vi "BuildRunScript.vi"(8 "ErrorArray In":errorcluster[](array[cluster]), 11 "NISTBus In":refnum<class "NISTBus.lvclass">) -> (0 "ErrorArray Out":errorcluster[](array[cluster]), 2 "Script":string[](array[string]), 3 "NISTBus Out":refnum<class "NISTBus.lvclass">)   [LabVIEW 2014, in "TestFramework.lvlib"]
uses:
  TestFramework.lvlib
  Bus/NISTBus.lvclass
  FGenModule/PublicAPI/Arguments/Broadcasts/clErrorRpt.ctl
  FGenPlugins/MyPluginBaseClass/TypeDef/PluginParams.ctl
  WfrmGenerator/WfrmModule/PublicAPI/Arguments/Broadcasts/clErrorRpt.ctl
  WfrmGenerator/WfrmModule/PublicAPI/Arguments/Requests/clLoadPlugin.ctl
  <vilib>/Utility/error.llb/Error Cluster From Error Code.vi
  <vilib>/ErrorRing/Error Ring.xnode
  FGenModule/FGenModule.lvlib
  <userlib>/NIST/NISTErrorLib/NISTErrorLib.lvlib
  WfrmGenerator/WfrmModule/WfrmModule.lvlib
  FGenPlugins/MyPluginBaseClass/NISTFGenPluginsBase.lvclass
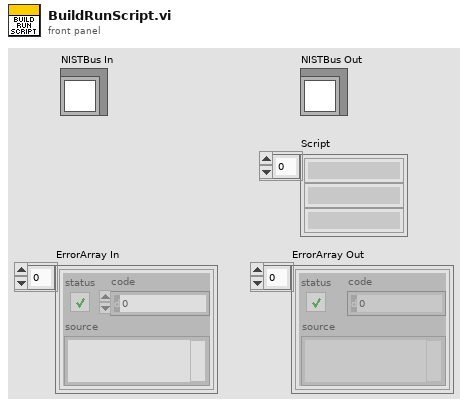
[diagram p1: front panel]
types:
  T1 = typedef "FGenModule.lvlib/clErrorRpt.ctl" = cluster{"error":errorcluster, "AdditionalInfo":string}
  T2 = typedef "WfrmModule.lvlib/clErrorRpt.ctl" = cluster{"error":errorcluster, "AdditionalInfo":string}
  T3 = typedef "WfrmModule.lvlib/clLoadPlugin.ctl" = cluster{"PathToPlugin":path}
  T4 = typedef "FGenModule.lvlib/clBroadcastEvents.ctl" = cluster{"DidInit":refnum<user-event>, "StatusUpdate":refnum<user-event>, "ErrorReport":refnum<user-event>, "DidStop":refnum<user-event>, "PathToINI":refnum<user-event>, "ChannelName":refnum<user-event>}
  T5 = typedef "FGenPlugins.lvlib/NISTFGenPluginsBase.lvclass/PluginParams.ctl" = cluster{"Path to Plugin INI":path}
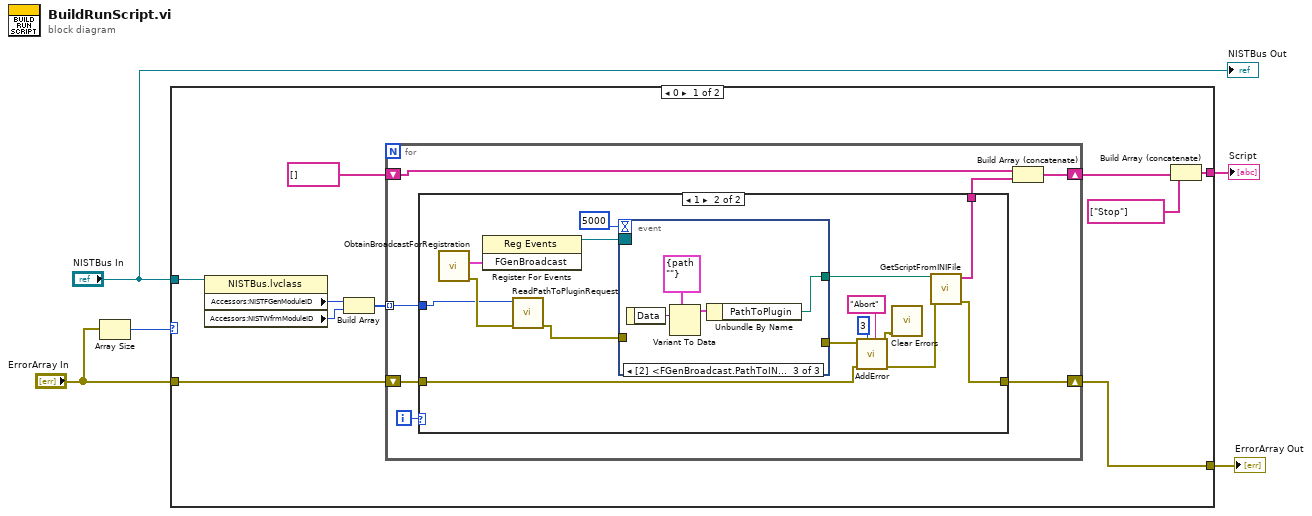
[diagram p0: block diagram]
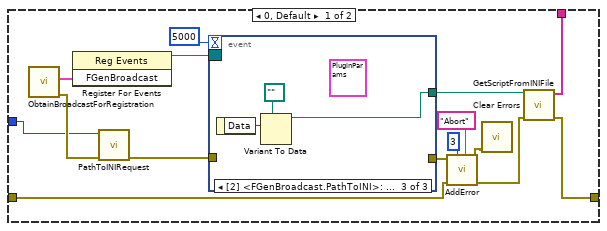
[diagram p2: hidden frame]
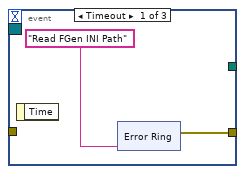
[diagram p3: hidden frame]
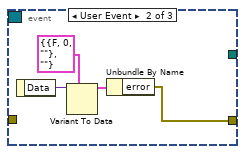
[diagram p4: hidden frame]
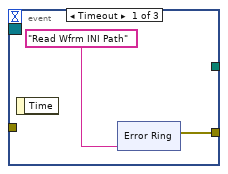
[diagram p5: hidden frame]
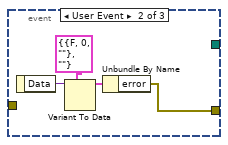
[diagram p6: hidden frame]
diagram:
  n1 = Array Size(array="ErrorArray In") -> (size(s)=w5:i32)
  n2 = case shown="0" w5 {
    tunnel: "ErrorArray In" -> [w10 w86]
    tunnel: "NISTBus In" -> [w15 _]
    tunnel: [w9 w86] -> w3
    tunnel: [w6 _] -> w2
    frame 0 {
      n3 = property class="NISTBus.lvclass"(reference=w15) -> ("Accessors:NISTFGenModuleID"=w14:i32, "Accessors:NISTWfrmModuleID"=w13:i32)  [unwired: 1 in, 2 out]
      n4 = Build Array(w14, w13) -> (w12:i32[])
      n5 = for {
        tunnel: w12 -> [w21] mode=indexing
        shift-right: [w18] -> w7
        shift-left: string[] [] -> [w17]
        shift-right: [w19] -> w9
        shift-left: w10 -> [w20]
        i -> [w22]
        n6 = case shown="1" w22 {
          tunnel: w21 -> [w27 w59]
          tunnel: w20 -> [w33 w64]
          tunnel: [w24 w55] -> w19
          tunnel: [w23 w54] -> w16
          frame 0, Default {
            n7 = call "ObtainBroadcastForRegistration.vi"() -> ("error out"=w29:errorcluster, "FGenBroadcast"=w37:T4)  [unwired: 10 in]
            n8 = register-events(w37) -> (reference out=w35:refnum<event-registration>)  [unwired: 2 in, 1 out]
            n9 = call "PathToINIRequest.vi"("error in (no error)"=w29, "ModuleID"=w27) -> ("error out"=w28:errorcluster)  [unwired: 9 in]
            n10 = event shown="[2] <FGenBroadcast.PathToINI>: User Event" {
              selector: w35 -> [_ _ _]
              dyn-events: _ -> [_ _ _]
              timeout: 5000 -> [_ _ _]
              tunnel: [w38 w47 _] -> w34
              tunnel: w28 -> [_ _ _]
              tunnel: [_ _ w51] -> w26
              event Timeout {
                n11 = event-data() -> ()  [unwired: 1 in, 1 out]
                n12 = xnode "Error Ring"("parameter 0"="Read FGen INI Path") -> ("error out"=w38:errorcluster)
              }
              event User Event {
                n13 = event-data() -> ("Data"=w50:variant)  [unwired: 1 in]
                n14 = Variant To Data(type=T1 {"error"={"status"=FALSE, "code"=0, "source"=""}, "AdditionalInfo"=""} ("Cluster"), Variant=w50) -> (data=w49:T1)  [unwired: 1 in, 1 out]
                n15 = Unbundle By Name(w49) -> ("error"=w47:errorcluster)
              }
              event User Event {
                (unwired) T5 {"Path to Plugin INI"=path "../../MyPlugins/Keysight335XX/Keysight335XX.ini"} ("PluginParams")
                n16 = event-data() -> ("Data"=w53:variant)  [unwired: 1 in]
                n17 = Variant To Data(type=path "" ("Path to Plugin INI"), Variant=w53) -> (data=w51:path)  [unwired: 1 in, 1 out]
              }
            }
            n18 = call <userlib>:"AddError.vi"("Severity"="Abort" ("String"), "Priority"=u8 3, "ErrorArray"=w33, "error in (no error)"=w34) -> ("ErrorArray"=w25:errorcluster[], "error out"=w30:errorcluster)  [unwired: 6 in]
            n19 = call <vilib>:"Clear Errors.vi"("error in (no error)"=w30) -> ()  [unwired: 5 in, 2 out]
            n20 = call "GetScriptFromINIFile.vi"("ErrorArray In"=w25, "Path"=w26) -> ("ErrorArray Out"=w24:errorcluster[], "Script"=w23:string[])  [unwired: 8 in]
          }
          frame 1 {
            n21 = call "ObtainBroadcastForRegistration.vi"() -> ("error out"=w60:errorcluster, "FGenBroadcast"=w68:T4)  [unwired: 10 in]
            n22 = register-events(w68) -> (reference out=w66:refnum<event-registration>)  [unwired: 2 in, 1 out]
            n23 = call "ReadPathToPluginRequest.vi"("error in (no error)"=w60, "ModuleID"=w59) -> ("error out"=w58:errorcluster)  [unwired: 9 in]
            n24 = event shown="[2] <FGenBroadcast.PathToINI>: User Event" {
              selector: w66 -> [_ _ _]
              dyn-events: _ -> [_ _ _]
              timeout: 5000 -> [_ _ _]
              tunnel: [w69 w78 _] -> w65
              tunnel: w58 -> [_ _ _]
              tunnel: [_ _ w82] -> w57
              event Timeout {
                n25 = event-data() -> ()  [unwired: 1 in, 1 out]
                n26 = xnode "Error Ring"("parameter 0"="Read Wfrm INI Path") -> ("error out"=w69:errorcluster)
              }
              event User Event {
                n27 = event-data() -> ("Data"=w81:variant)  [unwired: 1 in]
                n28 = Variant To Data(type=T2 {"error"={"status"=FALSE, "code"=0, "source"=""}, "AdditionalInfo"=""} ("Cluster"), Variant=w81) -> (data=w79:T2)  [unwired: 1 in, 1 out]
                n29 = Unbundle By Name(w79) -> ("error"=w78:errorcluster)
              }
              event User Event {
                n30 = event-data() -> ("Data"=w85:variant)  [unwired: 1 in]
                n31 = Variant To Data(type=T3 {"PathToPlugin"=path ""} ("clLoadPlugin"), Variant=w85) -> (data=w83:T3)  [unwired: 1 in, 1 out]
                n32 = Unbundle By Name(w83) -> ("PathToPlugin"=w82:path)
              }
            }
            n33 = call <userlib>:"AddError.vi"("Severity"="Abort" ("String"), "Priority"=u8 3, "ErrorArray"=w64, "error in (no error)"=w65) -> ("ErrorArray"=w56:errorcluster[], "error out"=w61:errorcluster)  [unwired: 6 in]
            n34 = call <vilib>:"Clear Errors.vi"("error in (no error)"=w61) -> ()  [unwired: 5 in, 2 out]
            n35 = call "GetScriptFromINIFile.vi"("ErrorArray In"=w56, "Path"=w57) -> ("ErrorArray Out"=w55:errorcluster[], "Script"=w54:string[])  [unwired: 8 in]
          }
        }
        n36 = Build Array (concatenate)(w17, w16) -> (w18:string[])
      }
      n37 = Build Array (concatenate)(w7, string[] ["Stop"]) -> (w6:string[])
    }
    frame 1, Default {
    }
  }
  "ErrorArray Out" <- w3
  "Script" <- w2
  "NISTBus Out" <- "NISTBus In"
